vi "Init.vi"(3 "Append These":refnum<class>[](array[class])) -> (1 "Action out":refnum<class "Act_Append Many.lvclass">)   [LabVIEW 2014, in "Act_Append Many.lvclass"]
uses:
  Act_Append Many.lvclass
  Act_Append Many.lvclass/Act_Append Many.ctl
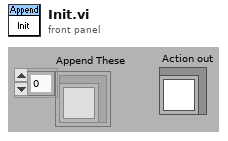
[diagram p1: front panel]
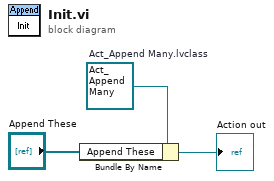
[diagram p0: block diagram]
diagram:
  w3 = refnum<class "Act_Append Many.lvclass"> refnum  # Act_Append Many.lvclass
  n1 = Bundle By Name(cluster=w3, "Append These"="Append These") -> (→"Action out":refnum<class "Act_Append Many.lvclass">)
